vi "Lookup Base Protocol Class.vi"(8 "error in (no error)":errorcluster, 10 "Protocol in":string, 11 "Class Lookup":variant) -> (0 "error out":errorcluster, 1 "Protocol out":T1, 2 "Protocol Parent out":refnum<class "Protocol Parent.lvclass">, 3 "Class Lookup out":variant)   [LabVIEW 2019, in "Instrument Addon Shared.lvlib"]
uses:
  Instrument Addon Shared.lvlib
  Support Libraries/Protocols/Protocols.lvlibp/Protocol Parent/Protocol Parent.lvclass
  Support Libraries/Protocols/Protocols.lvlibp/Protocol Parent/Types/Base Protocol Type.ctl
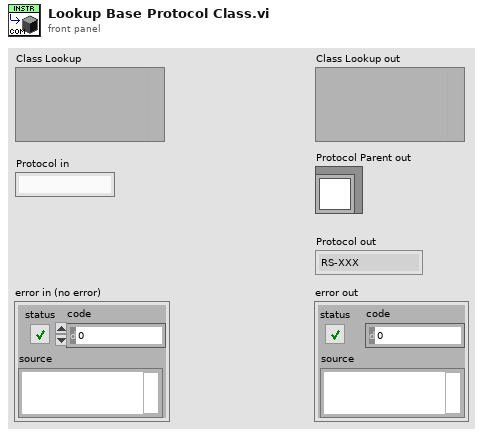
[diagram p1: front panel]
types:
  T1 = typedef "Protocols.lvlibp/Protocol Parent.lvclass/Base Protocol Type.ctl" = enum16{"RS-XXX", "VISA", "TCPIP", "UDP"}
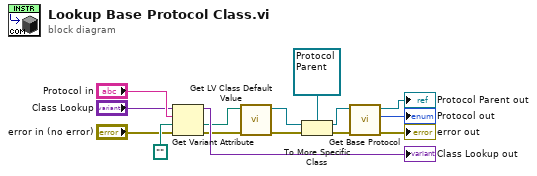
[diagram p0: block diagram]
diagram:
  n1 = Get Variant Attribute(Variant="Class Lookup", name="Protocol in", default value (empty Variant)=path "", error in="error in (no error)") -> (duplicate Variant=→"Class Lookup out":variant, value=w5:path, error out=w6:errorcluster)  [unwired: 1 out]
  n2 = call <vilib>:"Get LV Class Default Value.vi"("error in (no error)"=w6, "class path"=w5) -> ("error out"=w7:errorcluster, "object"=w10:refnum<class>)  [unwired: 8 in]
  n3 = To More Specific Class(target class=refnum<class "Protocol Parent.lvclass"> refnum ("Protocols.lvlibp:Protocol Parent.lvclass"), reference=w10, error in=w7) -> (specific class reference=w12:refnum<class "Protocol Parent.lvclass">, error out=w8:errorcluster)
  n4 = call-dynamic "Get Base Protocol.vi"("error in (no error)"=w8, "Protocol Parent in"=w12) -> ("error out"=→"error out":errorcluster, "Protocol out"=→"Protocol out":T1, "Protocol Parent out"=→"Protocol Parent out":refnum<class "Protocol Parent.lvclass">)  [unwired: 7 in]
